vi "Initiate Acquisition And Wait.vi"(8 "error in (no error)":errorcluster, 10 "Maximum Time (5000)":i32=5000, 11 "VISA resource name":refnum<visa-resource-name>) -> (0 "error out":errorcluster, 3 "VISA resource name out":refnum<visa-resource-name>)   [LabVIEW 2020, in "Rohde&Schwarz RTx Oscilloscopes.lvlib"]
doc: "This VI initiates a waveform acquisition and wits for it to finish\n\nAttribute:\nRSRTX_ATTR_RUN_SINGLE_WAIT_FOR_OPC\n\nRemote-control command:\nSINGle"
uses:
  Rohde&Schwarz RTx Oscilloscopes.lvlib
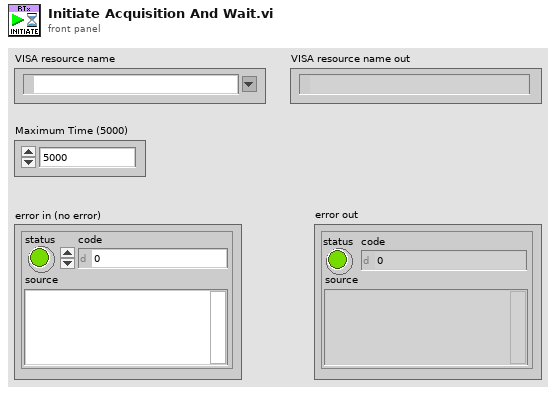
[diagram p1: front panel]
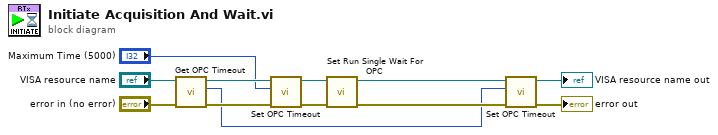
[diagram p0: block diagram]
diagram:
  n1 = call "Get OPC Timeout.vi"("error in (no error)"="error in (no error)", "VISA resource name"="VISA resource name") -> ("error out"=w12:errorcluster, "OPC Timeout"=w1:i32, "VISA resource name out"=w11:refnum<visa-resource-name>)  [unwired: 7 in]
  n2 = call "Set OPC Timeout.vi"("error in (no error)"=w12, "OPC Timeout"="Maximum Time (5000)", "VISA resource name"=w11) -> ("error out"=w10:errorcluster, "VISA resource name out"=w9:refnum<visa-resource-name>)  [unwired: 7 in]
  n3 = call "Set Run Single Wait For OPC"("error in (no error)"=w10, "instrument handle"=w9) -> ("error out"=w5:errorcluster, "instrument handle out"=w6:refnum<visa-resource-name>)  [unwired: 8 in]
  n4 = call "Set OPC Timeout.vi"("error in (no error)"=w5, "OPC Timeout"=w1, "VISA resource name"=w6) -> ("error out"=→"error out":errorcluster, "VISA resource name out"=→"VISA resource name out":refnum<visa-resource-name>)  [unwired: 7 in]
